vi "Project-1.vi"() -> ()   [LabVIEW 2024]
uses:
  <vilib>/express/express signal manip/GetorSetDDTAttributes/Set DDT Attributes/Set DDT Properties.xnode
  <vilib>/express/express shared/transition.llb/Dynamic To Waveform Array.vi
  <vilib>/express/express signal manip/GetorSetDDTAttributes/Set DDT Attributes/SetT0.vi
  <vilib>/express/express shared/transition.llb/Waveform Array To Dynamic.vi
  <vilib>/Utility/error.llb/DialogType.ctl
  <vilib>/DAQmx/create/channels.llb/DAQmx Create Channel (CI-Position-Angular Encoder).vi
  <vilib>/DAQmx/read.llb/DAQmx Read (Analog 1D Wfm NChan 1Samp).vi
panel:
  out "Waveform Graph 3":waveform(dbl)[](graph)
  in  "Decoding Type":i32(ring)=10092 items=["X1"=10090, "X2"=10091, "X4"=10092, "Two Pulse Counting"=10313]
  in  "Pulses per Revolution":u32=24
  in  "Z Index Phase":i32(ring)=10040 items=["A High B High"=10040, "A High B Low"=10041, "A Low B High"=10042, "A Low B Low"=10043]
  in  "Z Index Value":dbl
  in  "Z Index Enable":bool
  in  "Counter(s)":tag="Dev1/ctr0"
  in  "stop":bool
  in  "Calibration constan gyro 2":dbl=0.00980665 format="%#_13g"
  in  "Calibration constant gyro 1":dbl=0.00980665 format="%#_13g"
  out "Waveform Graph 2":dynamicdata(graph)
  out "Filename Out":path
  out "Saving Data":bool
  in  "Filename":path=path "test.lvm"
  in  "Enable":bool=TRUE
  out "raw accel":dynamicdata(graph)
  out "Waveform Graph":dynamicdata(graph)
  in  "timeout (s)":dbl=10.0 format="%0.2f"
  in  "Number of points to acquire":i32=100
  in  "Scan Rate":dbl=1000.0
  # "Project 1- Analog Data Acquisition and Digital Filtering\nCandela Solis and Armando Loynaz"
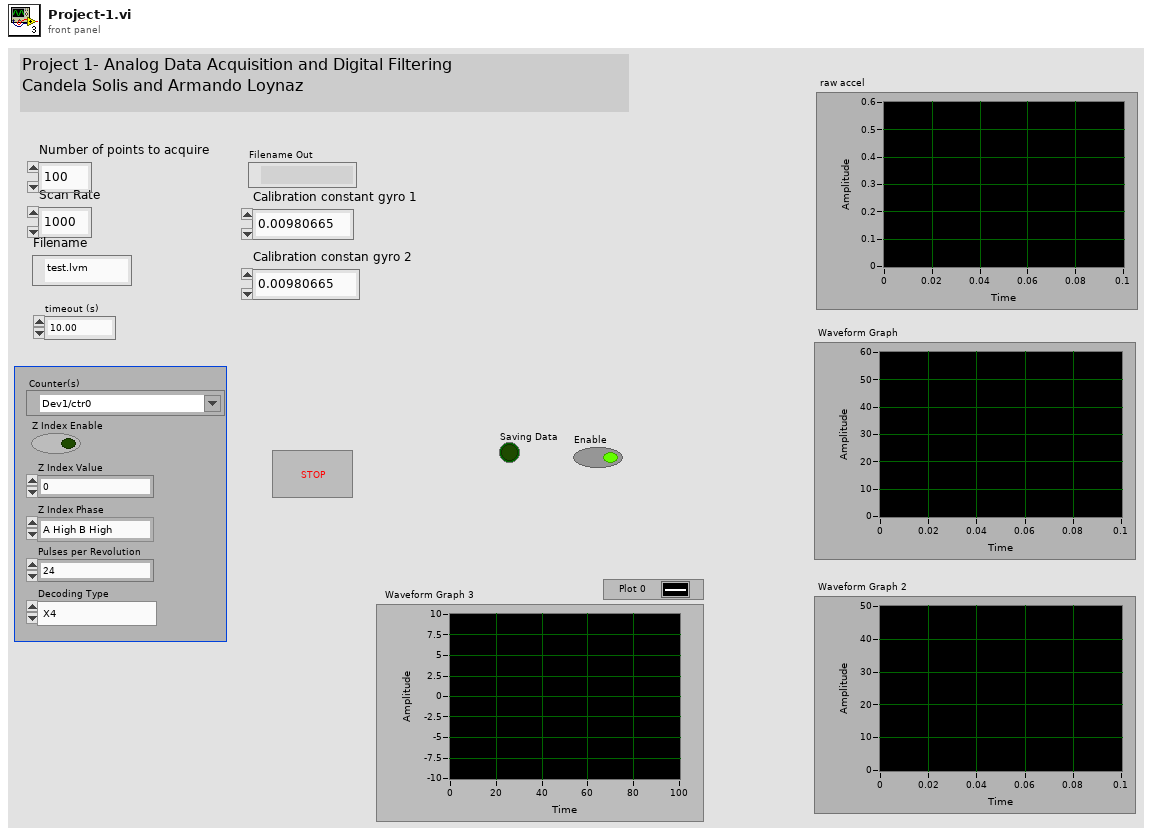
[diagram p1: front panel]
types:
  T1 = typedef "DialogType.ctl" = u16
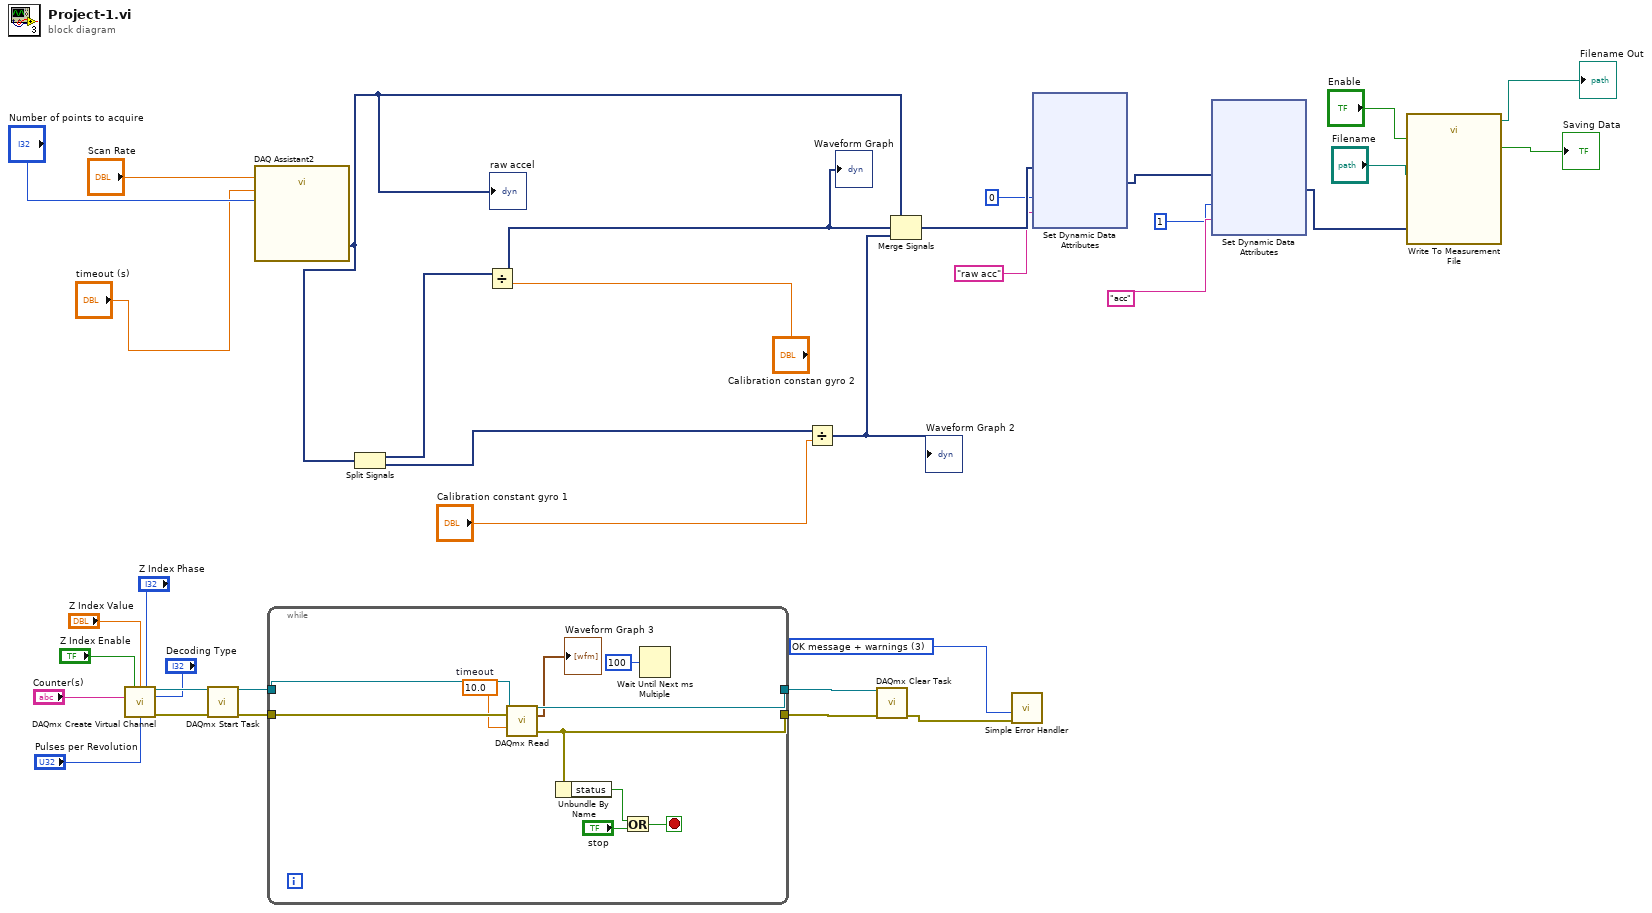
[diagram p0: block diagram]
diagram:
  w6 = T1 3 items=["no dialog", "OK message", "continue or stop message", "OK message + warnings", "continue/stop + warnings"] ("type of dialog (OK msg:1)")
  n1 = call-poly <vilib>:"DAQmx Create Virtual Channel.vi"("z index enable"="Z Index Enable", "z index value"="Z Index Value", "z index phase"="Z Index Phase", "counter"="Counter(s)", "decoding type"="Decoding Type", "pulses per revolution"="Pulses per Revolution") -> ("task out"=w8:refnum<k21>, "error out"=w9:errorcluster)  [unwired: 8 in]
  n2 = call <vilib>:"DAQmx Start Task.vi"("task/channels in"=w8, "error in"=w9) -> ("task out"=w11:refnum<k21>, "error out"=w14:errorcluster)  [unwired: 12 in]
  n3 = call "DAQ Assistant2"("rate"="Scan Rate", "number of samples"="Number of points to acquire", "timeout (s)"="timeout (s)") -> ("data"=w20:dynamicdata)  [unwired: 14 in, 2 out]
  "raw accel" <- w20
  n4 = while {
    tunnel: w14 -> [w45]
    tunnel: [w41] -> w13
    tunnel: w11 -> [w40]
    tunnel: [w39] -> w10
    stop <- w44 stop-if-true
    w38 = 10.0  # timeout
    n5 = call-poly <vilib>:"DAQmx Read.vi"("task/channels in"=w40, "timeout"=w38, "error in"=w45) -> ("task out"=w39:refnum<k21>, "data"=→"Waveform Graph 3":waveform(dbl)[], "error out"=w41:errorcluster)  [unwired: 10 in]
    n6 = Unbundle By Name(w41) -> ("status"=w42:bool)
    n7 = Or(x=w42, y="stop") -> (x .or. y?=w44:bool)
    n8 = Wait Until Next ms Multiple(millisecond multiple=u32 100) -> ()  [unwired: 1 out]
  }
  n9 = Split Signals(w20) -> (w17:dynamicdata, w16:dynamicdata)  [unwired: 2 in]
  n10 = Divide(x=w17, y="Calibration constan gyro 2") -> (x/y=w19:dynamicdata)
  "Waveform Graph" <- w19
  n11 = Divide(x=w16, y="Calibration constant gyro 1") -> (x/y=w15:dynamicdata)
  "Waveform Graph 2" <- w15
  n12 = call <vilib>:"DAQmx Clear Task.vi"("task in"=w10, "error in"=w13) -> ("error out"=w12:errorcluster)  [unwired: 13 in]
  n13 = Merge Signals(w20, w19, w15) -> (w31:dynamicdata)
  n14 = call <vilib>:"Simple Error Handler.vi"("type of dialog (OK msg:1)"=w6, "error in (no error)"=w12) -> ()  [unwired: 3 in, 5 out]
  n15 = xnode "Set Dynamic Data Attributes"("Signals In"=w31, "Signal Index"=0, "Signal Name"="raw acc") -> ("Signals Out"=w28:dynamicdata)  [unwired: 1 in, 1 out]
  n16 = xnode "Set Dynamic Data Attributes"("Signals In"=w28, "Signal Index"=1, "Signal Name"="acc") -> ("Signals Out"=w25:dynamicdata)  [unwired: 1 in, 1 out]
  n17 = call "Write To Measurement File"("Signals"=w25, "Enable"="Enable", "Filename"="Filename") -> ("Filename Out"=→"Filename Out":path, "Saving Data"=→"Saving Data":bool)  [unwired: 14 in, 1 out]
